vi "子窗口VI.vi"() -> ()   [LabVIEW 2012]
panel:
  in  "停止":bool
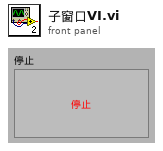
[diagram p1: front panel]
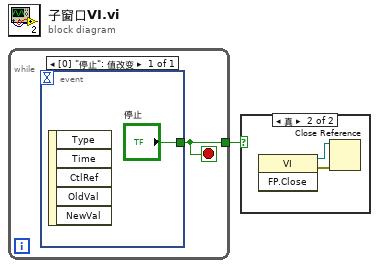
[diagram p0: block diagram]
diagram:
  n1 = while {
    tunnel: [w2] -> w1
    stop <- w2 stop-if-true
    n2 = event shown="[0] \"停止\": 值改变" {
      selector: _ -> [_]
      dyn-events: _ -> [_]
      timeout: _ -> [_]
      tunnel: ["停止"] -> w2
      event "停止": Value Change {
        n3 = event-data() -> ()  [unwired: 1 in, 5 out]
      }
    }
  }
  n4 = case shown="真" w1 {
    frame False {
    }
    frame True {
      n5 = invoke class="VI" method="FP.Close"() -> (reference out=w4:refnum<vi>, error out=w5:errorcluster)  [unwired: 3 in, 1 out]
      n6 = Close Reference(reference=w4, error in (no error)=w5) -> ()  [unwired: 1 out]
    }
  }
